vi "Measurement_Settings.vi"(3 "error in":errorcluster) -> ()   [LabVIEW 2011]
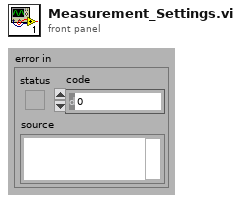
[diagram p1: front panel]
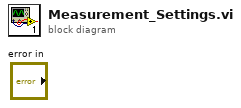
[diagram p0: block diagram]
diagram:
